vi "VI-Get Typedef Controls.vi"(0 "Path to typdef":path, 11 "error in (no error)":errorcluster) -> (4 "Controls[]":refnum<vi>[](array[refnum]), 15 "error out":errorcluster)   [LabVIEW 2015]
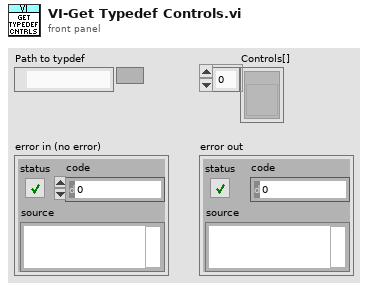
[diagram p1: front panel]
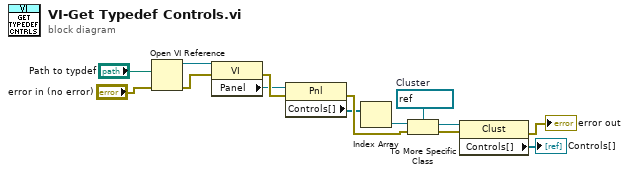
[diagram p0: block diagram]
diagram:
  w3 = refnum<vi> refnum  # Cluster
  n1 = Open VI Reference(vi path="Path to typdef", error in (no error)="error in (no error)") -> (vi reference=w7:refnum<vi>, error out=w10:errorcluster)  [unwired: 4 in]
  n2 = property class="VI"(reference=w7, error in=w10) -> (error out=w11:errorcluster, "Panel"=w6:refnum<vi>)  [unwired: 1 out]
  n3 = property class="Pnl"(reference=w6, error in=w11) -> (error out=w12:errorcluster, "Controls[]"=w5:refnum<vi>[])  [unwired: 1 out]
  n4 = Index Array(array=w5) -> (element=w4:refnum<vi>)  [unwired: 1 in]
  n5 = To More Specific Class(target class=w3, reference=w4, error in=w12) -> (specific class reference=w2:refnum<vi>, error out=w13:errorcluster)
  n6 = property class="Clust"(reference=w2, error in=w13) -> (error out=→"error out":errorcluster, "Controls[]"=→"Controls[]":refnum<vi>[])  [unwired: 1 out]
